vi "GetChanContents.vi"(8 "error in":errorcluster, 11 "ChanGrp.lvclass":refnum<class "ChanGrp.lvclass">) -> (0 "error out":errorcluster, 1 "Num of Chans":i32, 2 "Multi Rate Mods in Grp":T1, 3 "All GrpChan Names":string[](array[string]), 4 "Chans w/ Modbus":i32[](array[numeric]), 5 "Chan Aliases":string[][](array[string]), 6 "Num Modbus Enbld":i16)   [LabVIEW 2012, in "Configuration Grandmaster.lvlib" / "ChanGrp.lvclass"]
uses:
  ChanGrp.lvclass
  SubVIs Main/SubVIs Build Grp/Custom Ctrls Bld/ge_MultiRateMods.ctl
  ChanGrp.lvclass/ChanGrp.ctl
  Measurements/Class Channel/Read Device.vi
  Measurements/Class Channel/Read ChanName.vi
  Measurements/Class Channel/Read Alias.vi
  Measurements/Class Channel/Read ModbusAddr.vi
  Measurements/Class Channel/Read ToModBus.vi
  Measurements/Class Channel/Channel.lvclass
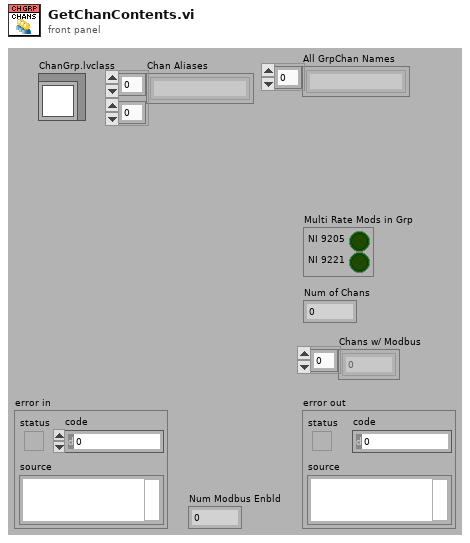
[diagram p1: front panel]
types:
  T1 = typedef "ge_MultiRateMods.ctl" = cluster{"NI 9205":bool, "NI 9221":bool}
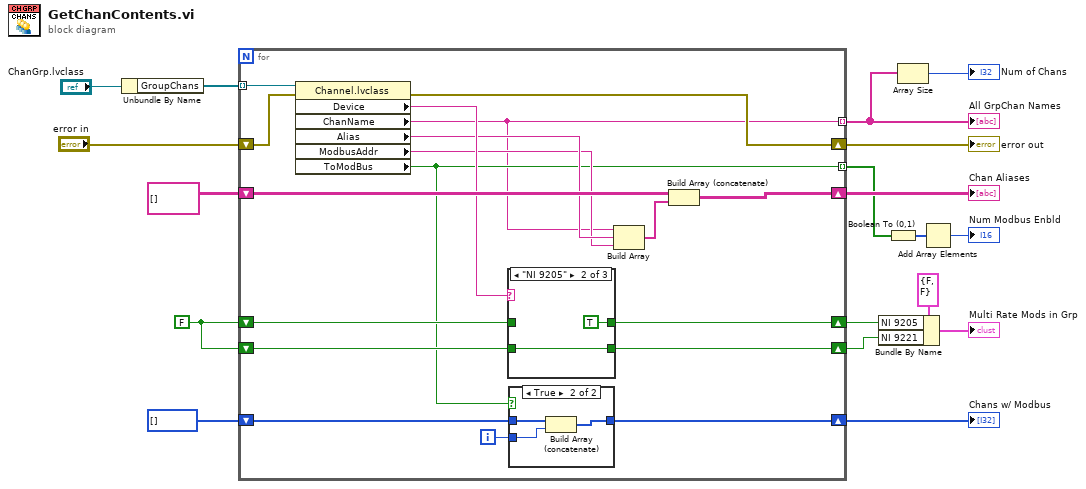
[diagram p0: block diagram]
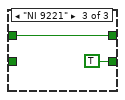
[diagram p4: hidden frame]
diagram:
  w17 = FALSE
  n1 = Unbundle By Name("ChanGrp.lvclass") -> ("GroupChans"=w7:refnum<class "Channel.lvclass">[])
  n2 = for {
    tunnel: w7 -> [w26] mode=indexing
    shift-right: [w34] -> w16
    shift-left: w17 -> [w36]
    shift-right: [w33] -> w15
    shift-left: w17 -> [w35]
    shift-right: [w30] -> w11
    shift-left: i32[] [] -> [w32]
    shift-right: [w27] -> w9
    shift-left: string[][] [] -> [w29]
    tunnel: [w19] -> w6 mode=indexing
    shift-right: [w21] -> w4
    shift-left: "error in" -> [w22]
    tunnel: [w20] -> w2 mode=indexing
    i -> [w31]
    n3 = property class="Channel.lvclass"(reference=w26, error in=w22) -> (error out=w21:errorcluster, "Device"=w25:string, "ChanName"=w19:string, "Alias"=w24:string, "ModbusAddr"=w23:string, "ToModBus"=w20:bool)  [unwired: 1 out]
    n4 = case shown="\"NI 9205\"" w25 {
      tunnel: w36 -> [w42 _ w46]
      tunnel: w35 -> [w41 w43 _]
      tunnel: [w42 TRUE w46] -> w34
      tunnel: [w41 w43 TRUE] -> w33
      frame Default {
      }
      frame "NI 9205" {
      }
      frame "NI 9221" {
      }
    }
    n5 = case shown="True" w20 {
      tunnel: w32 -> [w37 w40]
      tunnel: w31 -> [_ w39]
      tunnel: [w37 w38] -> w30
      frame False {
      }
      frame True {
        n6 = Build Array (concatenate)(w40, w39) -> (w38:i32[])
      }
    }
    n7 = Build Array(w19, w24, w23) -> (w28:string[])
    n8 = Build Array (concatenate)(w29, w28) -> (w27:string[][])
  }
  "Chans w/ Modbus" <- w11
  "Chan Aliases" <- w9
  "All GrpChan Names" <- w6
  "error out" <- w4
  n9 = Bundle By Name(cluster=T1 {"NI 9205"=FALSE, "NI 9221"=FALSE} ("Multi Rate Mods in Grp"), "NI 9205"=w16, "NI 9221"=w15) -> (→"Multi Rate Mods in Grp":T1)
  n10 = Boolean To (0,1)(Boolean=w2) -> (0, 1=w3:i16[])
  n11 = Array Size(array=w6) -> (size(s)=→"Num of Chans":i32)
  n12 = Add Array Elements(numeric array=w3) -> (sum=→"Num Modbus Enbld":i16)
